vi "StartAcquisition.vi"(8 "error in":errorcluster, 11 "camera handle in":u64) -> (0 "error out":errorcluster, 3 "camera handle out":u64)   [LabVIEW 2014, in "PICam.lvlib"]
doc: "PicamAdcAnalogGain is the set of electronic gain settings for pixel digitization.\n\nPicamAdcAnalogGain_Low Small amplification.\nPicamAdcAnalogGain_Medium Average amplification.\nPicamAdcAnalogGain_High Large amplification.\n\nRefer to the user manual for the specific\ncamera being used for complete information."
uses:
  PICam.lvlib
  Picam32.dll
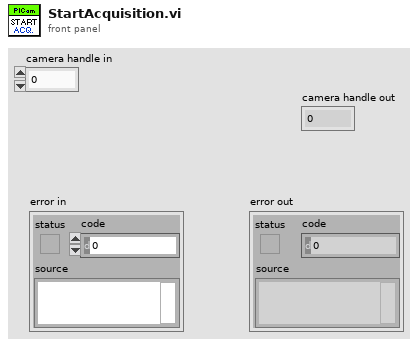
[diagram p1: front panel]
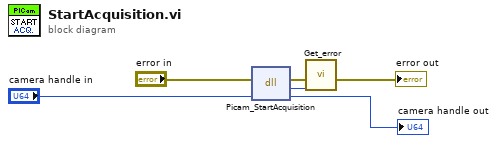
[diagram p0: block diagram]
diagram:
  n1 = dll-call lib="Picam32.dll" fn="Picam_StartAcquisition"(error in="error in", "camera"="camera handle in") -> (error out=w6:errorcluster, "return type"=w5:i32, "camera"=→"camera handle out":u64)  [unwired: 2 in, 1 out]
  n2 = call "Get_error.vi"("PICam_Error"=w5, "error in (no error)"=w6) -> ("error out"=→"error out":errorcluster)  [unwired: 9 in]
